vi "例7.9使用属性节点控制屏幕的初始化和指示灯的闪烁.vi"() -> ()   [LabVIEW 2017]
panel:
  out "布尔":bool
  out "波形图表":dbl(graph)
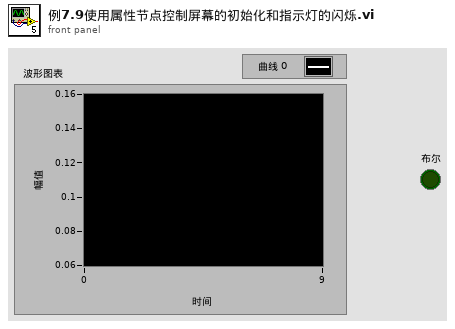
[diagram p1: front panel]
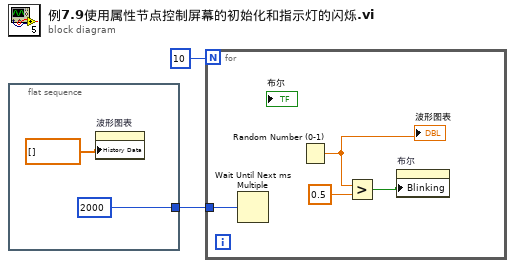
[diagram p0: block diagram]
diagram:
  n1 = flat-sequence {
    tunnel: [2000] -> w1
    frame #0 {
      n2 = property on="波形图表" class="WFChart (严格)"("History Data"=dbl[] [] ("历史数据")) -> ()  [unwired: 2 in, 2 out]
    }
  }
  n3 = for {
    N: 10 -> [_]
    tunnel: w1 -> [w5]
    n4 = Wait Until Next ms Multiple(millisecond multiple=w5) -> ()  [unwired: 1 out]
    n5 = Random Number (0-1)() -> (number: 0 to 1=w8:dbl)
    "波形图表" <- w8
    n6 = Greater?(x=w8, y=0.5) -> (0:w6:bool)
    n7 = property on="布尔" class="Bool (严格)"("Blinking"=w6) -> ()  [unwired: 2 in, 2 out]
  }
